vi "test - prealloc.vi"() -> ()   [LabVIEW 2022 SP3]
panel:
  in  "Slide":dbl(slide) scale=0.0..10.0
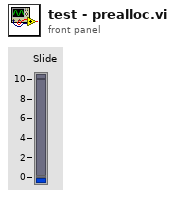
[diagram p1: front panel]
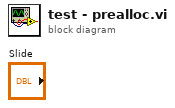
[diagram p0: block diagram]
diagram:
